vi "open.vi"(2 "serialName":string, 3 "Error In":errorcluster caption="错误输入") -> (0 "返回类型":i32, 1 "Error Out":errorcluster caption="错误输出")   [LabVIEW 2013, in "EM_CVx.lvlib"]
uses:
  EM_CVx.lvlib
  library/moverLibrary_x86.dll
  library/moverLibrary_x64.dll
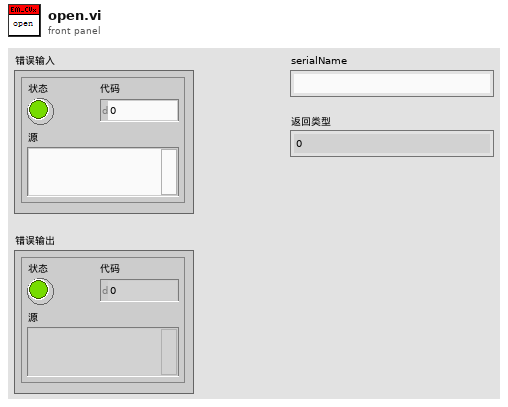
[diagram p1: front panel]
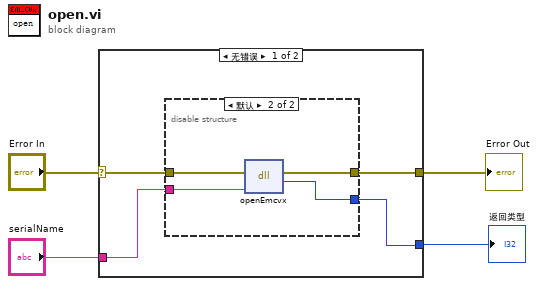
[diagram p0: block diagram]
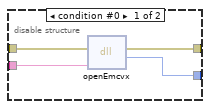
[diagram p2: hidden frame]
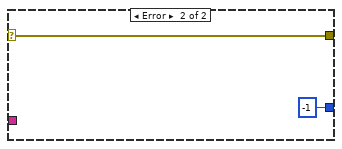
[diagram p3: hidden frame]
diagram:
  n1 = case shown="无错误" "Error In" {
    selector: "Error In" -> [w7 w18]
    tunnel: "serialName" -> [w8 _]
    tunnel: [w6 w18] -> w1
    tunnel: [w5 -1 ("返回类型")] -> w2
    frame No Error {
      n2 = disable-structure shown="默认" {
        disable-tunnel: w7 -> [w12 w16]
        disable-tunnel: w8 -> [w11 w15]
        disable-tunnel: [w10 w13] -> w6
        disable-tunnel: [w9 w14] -> w5
        frame condition #0 {
          n3 = dll-call lib="E:/5-mover/4-labView/EM_CVx_2013/library/moverLibrary_x64.dll" fn="openEmcvx"(error in=w12, "serialName"=w11) -> (error out=w10:errorcluster, "返回类型"=w9:i32)  [unwired: 3 in, 1 out]
        }
        frame condition #1 (active) {
          n4 = dll-call lib="E:/5-mover/4-labView/EM_CVx_2013/library/moverLibrary_x86.dll" fn="openEmcvx"(error in=w16, "serialName"=w15) -> (error out=w13:errorcluster, "返回类型"=w14:i32)  [unwired: 3 in, 1 out]
        }
      }
    }
    frame Error {
    }
  }
  "返回类型" <- w2
  "Error Out" <- w1
